vi "API Rcv Data Init.vi"(2 "错误输入（无错误）":errorcluster) -> (0 "错误输出":errorcluster, 1 "RTV":bool)   [LabVIEW 2011, in "API DYM.lvlib"]
uses:
  API DYM.lvlib
  DyMechnicalPlatform.dll
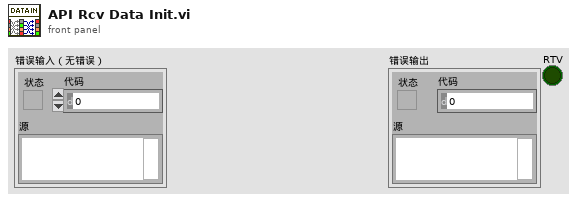
[diagram p1: front panel]
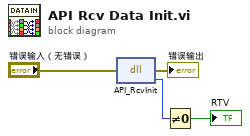
[diagram p0: block diagram]
diagram:
  n1 = dll-call lib="D:/Documents/GitHub/DYSYS/DYSYS/API/DyMechnicalPlatform.dll" fn="API_RcvInit"(error in="错误输入（无错误）") -> (error out=→"错误输出":errorcluster, "RTV"=w2:i32)  [unwired: 2 in, 1 out]
  n2 = Not Equal To 0?(x=w2) -> (x != 0?=→"RTV":bool)
